vi "Threshold.vi"(8 "sign":bool=TRUE, 10 "Multiplier":dbl min=-2.0 max=0.0 step=1.0, 11 "Slide":dbl(slide) min=0.0 max=9.0 step=1.0 scale=0.0..9.0 scale format="%#_2g") -> (3 "New Threshold":dbl)   [LabVIEW 2013]
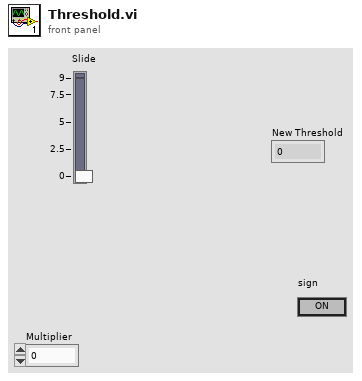
[diagram p1: front panel]
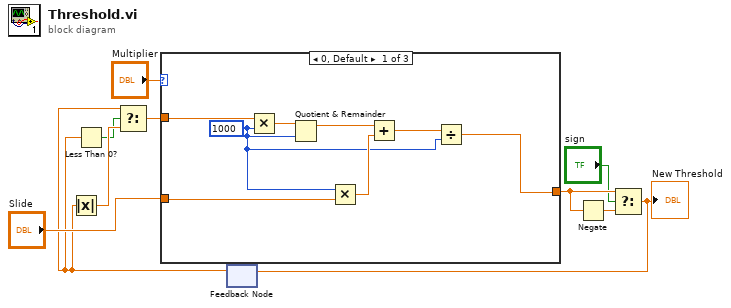
[diagram p0: block diagram]
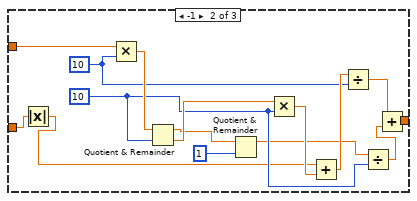
[diagram p2: hidden frame]
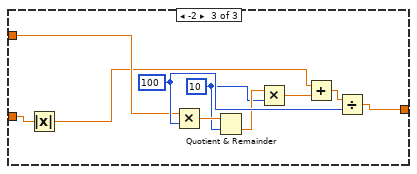
[diagram p3: hidden frame]
diagram:
  n1 = feedback #1() -> (w2:dbl)  [unwired: 1 in]
  n2 = Absolute Value(x=w2) -> (abs(x)=w8:dbl)
  n3 = Less Than 0?(x=w2) -> (x < 0?=w1:bool)
  n4 = Select(t=w2, s=w1, f=w8) -> (s? t:f=w9:dbl)
  n5 = case shown="0, Default" "Multiplier" {
    tunnel: "Slide" -> [w13 w20 w35]
    tunnel: w9 -> [w12 w28 w37]
    tunnel: [w11 w26 w36] -> w6
    frame 0, Default {
      w14 = 1000
      n6 = Multiply(x=w12, y=w14) -> (x*y=w18:dbl)
      n7 = Quotient & Remainder(x=w18, y=w14) -> (x-y*floor(x/y)=w17:dbl)  [unwired: 1 out]
      n8 = Multiply(x=w14, y=w13) -> (x*y=w16:dbl)
      n9 = Add(x=w17, y=w16) -> (x+y=w15:dbl)
      n10 = Divide(x=w15, y=w14) -> (x/y=w11:dbl)
    }
    frame -1 {
      w23 = 10
      w31 = 10
      n11 = Absolute Value(x=w20) -> (abs(x)=w19:dbl)
      n12 = Multiply(x=w28, y=w31) -> (x*y=w33:dbl)
      n13 = Quotient & Remainder(x=w33, y=w23) -> (x-y*floor(x/y)=w24:dbl, floor(x/y)=w30:dbl)
      n14 = Quotient & Remainder(x=w24, y=1) -> (x-y*floor(x/y)=w22:dbl)  [unwired: 1 out]
      n15 = Multiply(x=w30, y=w23) -> (x*y=w29:dbl)
      n16 = Add(x=w19, y=w29) -> (x+y=w32:dbl)
      n17 = Divide(x=w32, y=w31) -> (x/y=w27:dbl)
      n18 = Divide(x=w22, y=w23) -> (x/y=w21:dbl)
      n19 = Add(x=w27, y=w21) -> (x+y=w26:dbl)
    }
    frame -2 {
      w39 = 10
      w41 = 100
      n20 = Absolute Value(x=w35) -> (abs(x)=w34:dbl)
      n21 = Multiply(x=w37, y=w41) -> (x*y=w43:dbl)
      n22 = Quotient & Remainder(x=w43, y=w39) -> (floor(x/y)=w40:dbl)  [unwired: 1 out]
      n23 = Multiply(x=w40, y=w39) -> (x*y=w38:dbl)
      n24 = Add(x=w34, y=w38) -> (x+y=w42:dbl)
      n25 = Divide(x=w42, y=w41) -> (x/y=w36:dbl)
    }
  }
  n26 = Negate(x=w6) -> (-x=w7:dbl)
  n27 = Select(t=w6, s="sign", f=w7) -> (s? t:f=w5:dbl)
  "New Threshold" <- w5
  n28 = feedback-in #1(w5) -> ()
